vi "RunScript.vi"(8 "ErrorArray In":errorcluster[](array[cluster]), 10 "Script":string[](array[string]), 11 "NISTBus In":refnum<class "NISTBus.lvclass">) -> (0 "ErrorArray Out":errorcluster[](array[cluster]), 2 "Data Out":variant, 3 "NISTBus Out":refnum<class "NISTBus.lvclass">)   [LabVIEW 2014, in "Bus.lvlib" / "NISTBus.lvclass"]
uses:
  NISTBus.lvclass
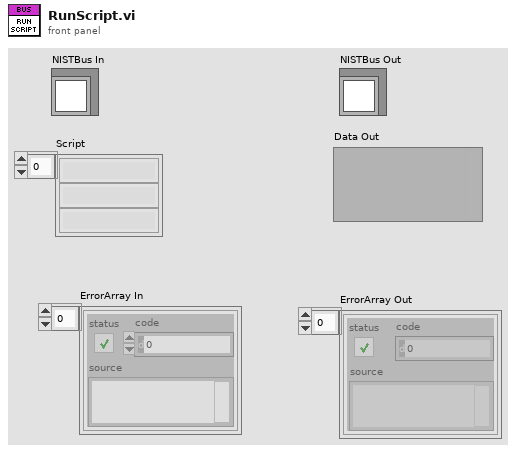
[diagram p1: front panel]
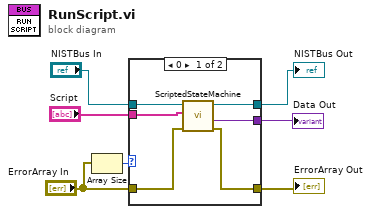
[diagram p0: block diagram]
diagram:
  n1 = Array Size(array="ErrorArray In") -> (size(s)=w7:i32)
  n2 = case shown="0" w7 {
    tunnel: "ErrorArray In" -> [w9 w15]
    tunnel: [w10 w15] -> w5
    tunnel: "NISTBus In" -> [w13 w14]
    tunnel: [w12 w14] -> w3
    tunnel: [w11 _] -> w2
    tunnel: "Script" -> [w8 _]
    frame 0 {
      n3 = call "ScriptedStateMachine.vi"("ErrorArray In"=w9, "Script"=w8, "NISTBus In"=w13) -> ("ErrorArray Out"=w10:errorcluster[], "Data Out"=w11:variant, "NISTBus Out"=w12:refnum<class "NISTBus.lvclass">)  [unwired: 6 in]
    }
    frame 1, Default {
    }
  }
  "Data Out" <- w2
  "NISTBus Out" <- w3
  "ErrorArray Out" <- w5
